vi "Set 1D Array String.vi"(5 "use temporary file?":bool, 8 "error in":errorcluster, 9 "value":string[](array[string]), 10 "variable name":string, 11 "GOLPI ref. in":T1={"pipe handle"={"lv_proc.dll file path"=path "", "process instance handle"=[]}, "fast read timeout [ms]"=500, "fast read settle time [ms]"=10, "fast read to multiple [ms]"=1, "max elements per input line"=100}) -> (0 "error out":errorcluster, 3 "GOLPI ref. out":T1={"pipe handle"={"lv_proc.dll file path"=path "", "process instance handle"=[]}, "fast read timeout [ms]"=500, "fast read settle time [ms]"=10, "fast read to multiple [ms]"=1, "max elements per input line"=100})   [LabVIEW 2013, in "GOLPI library.lvlib"]
uses:
  GOLPI library.lvlib
  Type Definitions/GOLPI reference Type Def.ctl
  LV Process.lvlibp/Pipe Handle.ctl
  LV Process.lvlibp
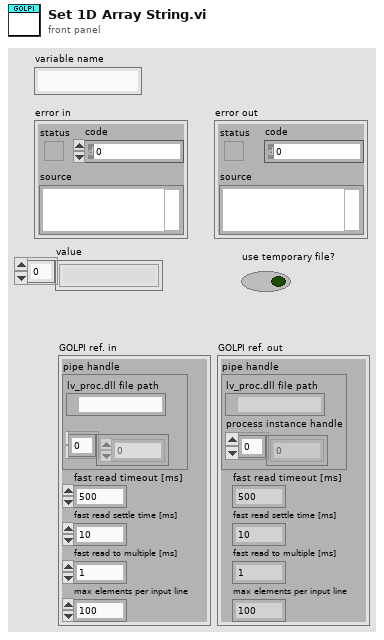
[diagram p1: front panel]
types:
  T1 = typedef "GOLPI library.lvlib/GOLPI reference Type Def.ctl" = cluster{"pipe handle":T2, "fast read timeout [ms]":u32, "fast read settle time [ms]":u32, "fast read to multiple [ms]":u32, "max elements per input line":u32}
  T2 = typedef "LV Process.lvlibp/Pipe Handle.ctl" = cluster{"lv_proc.dll file path":path, "process instance handle":u32[]}
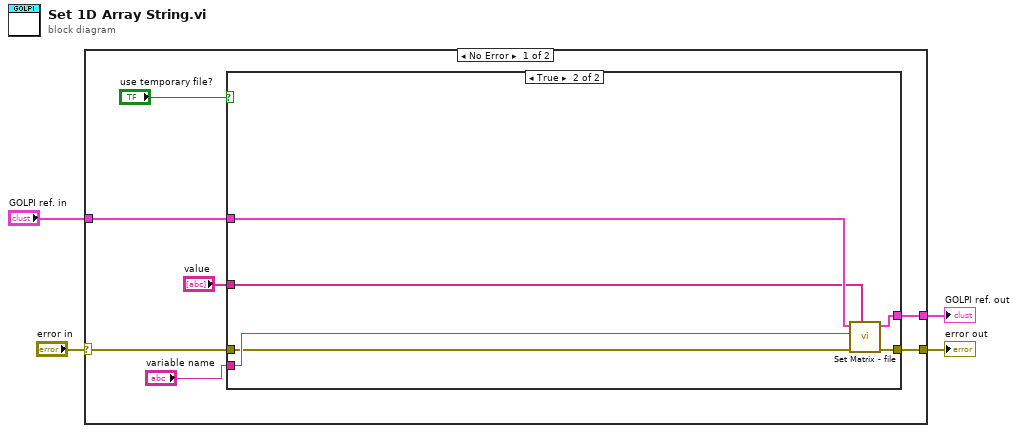
[diagram p0: block diagram]
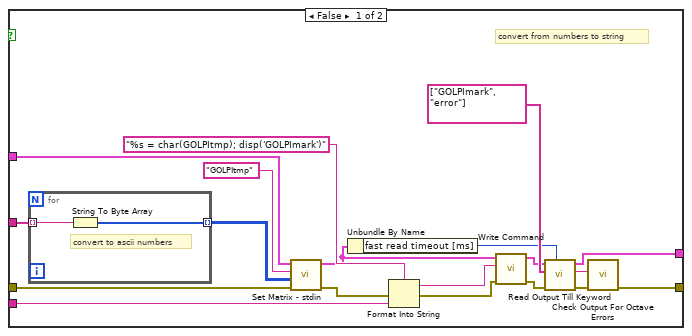
[diagram p2: hidden frame]
diagram:
  n1 = case shown="No Error" "error in" {
    selector: "error in" -> [w7 w40]
    tunnel: [w11 w40] -> w4
    tunnel: "GOLPI ref. in" -> [w6 w39]
    tunnel: [w10 w39] -> w1
    frame No Error {
      n2 = case shown="True" "use temporary file?" {
        tunnel: [w30 w35] -> w11
        tunnel: [w29 w34] -> w10
        tunnel: "variable name" -> [w27 w38]
        tunnel: "value" -> [w13 w33]
        tunnel: w7 -> [w17 w36]
        tunnel: w6 -> [w16 w37]
        frame False {
          # "convert from numbers to string"
          n3 = for {
            tunnel: w13 -> [w32] mode=indexing
            tunnel: [w31] -> w12 mode=indexing
            # "convert to ascii numbers"
            n4 = String To Byte Array(string=w32) -> (unsigned byte array=w31:u8[])
          }
          n5 = call "Set Matrix - stdin.vi"("error in"=w17, "value"=w12, "variable name"="GOLPItmp", "GOLPI ref. in"=w16) -> ("error out"=w15:errorcluster, "GOLPI ref. out"=w14:T1)  [unwired: 6 in]
          n6 = Unbundle By Name(w14) -> ("fast read timeout [ms]"=w19:u32)
          n7 = Format Into String(format string="%s = char(GOLPItmp); disp('GOLPImark')", error in=w15, w27) -> (resulting string=w25:string, error out=w26:errorcluster)  [unwired: 1 in]
          n8 = call "Write Command.vi"("error in"=w26, "command"=w25, "GOLPI ref. in"=w14) -> ("error out"=w24:errorcluster, "GOLPI ref. out"=w21:T1)  [unwired: 7 in]
          n9 = call "Read Output Till Keyword.vi"("timeout [ms]"=w19, "error in"=w24, "keywords"=string[] ["GOLPImark", "error"], "GOLPI ref. in"=w21) -> ("error out"=w23:errorcluster, "read buffer"=w20:string, "GOLPI ref. out"=w29:T1)  [unwired: 4 in, 1 out]
          n10 = call "Check Output For Octave Errors.vi"("error in"=w23, "read buffer"=w20) -> ("error out"=w30:errorcluster)  [unwired: 9 in]
        }
        frame True {
          n11 = call "Set Matrix - file.vi"("string array"=w33, "error in (no error)"=w36, "variable name"=w38, "GOLPI ref. in"=w37) -> ("error out"=w35:errorcluster, "GOLPI ref. out"=w34:T1)  [unwired: 6 in]
        }
      }
    }
    frame Error {
    }
  }
  "error out" <- w4
  "GOLPI ref. out" <- w1
